vi "Calculate Directory Size.vi"(1 "Directory":string, 2 "Directory Tree":T1) -> (0 "Directory Size":u64)   [LabVIEW 2020, in "AoC 2022.lvlib"]
uses:
  AoC 2022.lvlib
  Directory Tree.ctl
  Directory Contents.ctl
  File.ctl
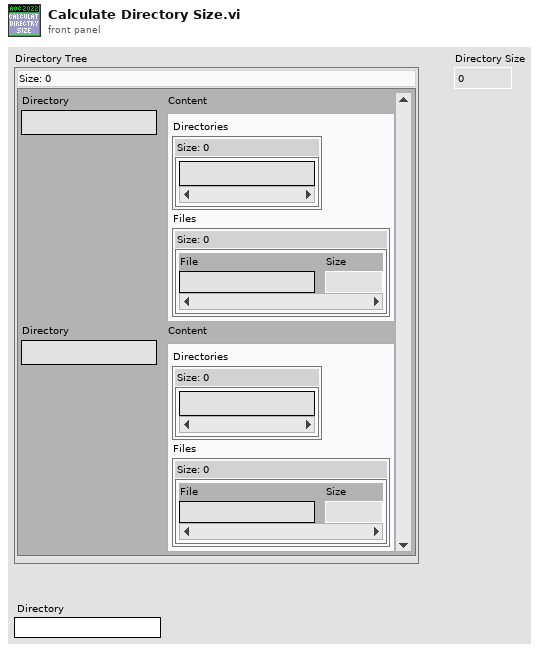
[diagram p1: front panel]
types:
  T1 = typedef "AoC 2022.lvlib/Directory Tree.ctl" = map{string, T2}
  T2 = typedef "AoC 2022.lvlib/Directory Contents.ctl" = cluster{"Directories":set{string}, "Files":T3}
  T3 = typedef "AoC 2022.lvlib/File.ctl" = map{string, u64}
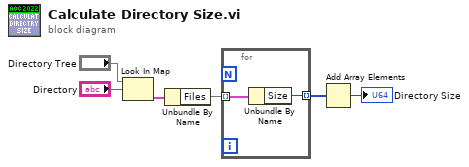
[diagram p0: block diagram]
diagram:
  n1 = Look In Map(map="Directory Tree", key="Directory") -> (value=w3:T2)  [unwired: 1 in, 1 out]
  n2 = Unbundle By Name(w3) -> ("Files"=w2:T3)
  n3 = for {
    tunnel: w2 -> [w8] mode=indexing
    tunnel: [w7] -> w1 mode=indexing
    n4 = Unbundle By Name(w8) -> ("Size"=w7:u64)
  }
  n5 = Add Array Elements(numeric array=w1) -> (sum=→"Directory Size":u64)
